vi "SendCmd.vi"(9 "cmd":string, 10 "exe":string="D:\\Program Files\\MVTec\\HALCON-17.12-Progress\\bin\\x64-win64\\hdevelop.exe") -> (0 "error out":errorcluster caption="错误输出", 1 "standard output":string, 2 "return code":i32 caption="返回代码", 3 "standard error":string)   [LabVIEW 2017]
panel:
  out "returnCode":string
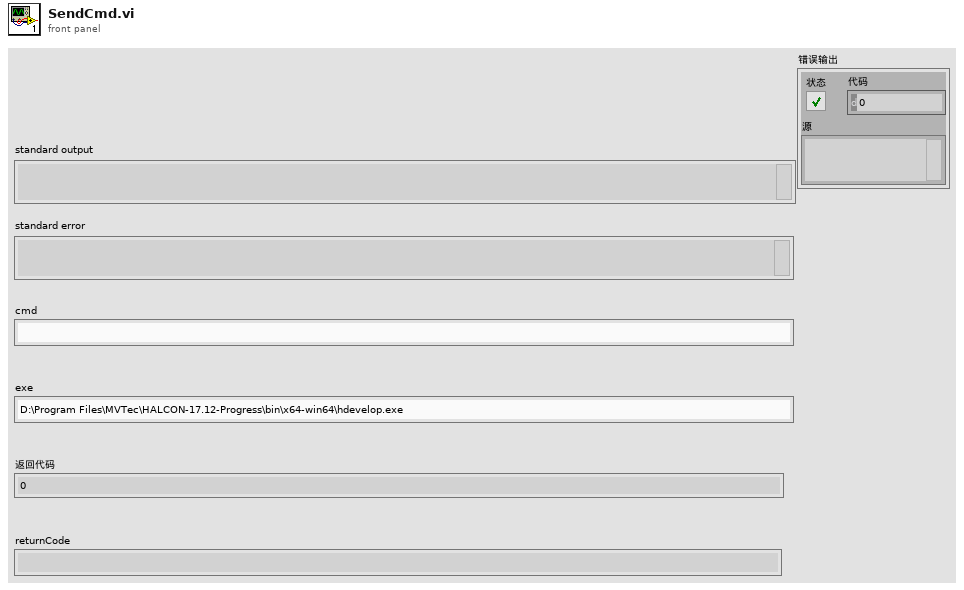
[diagram p1: front panel]
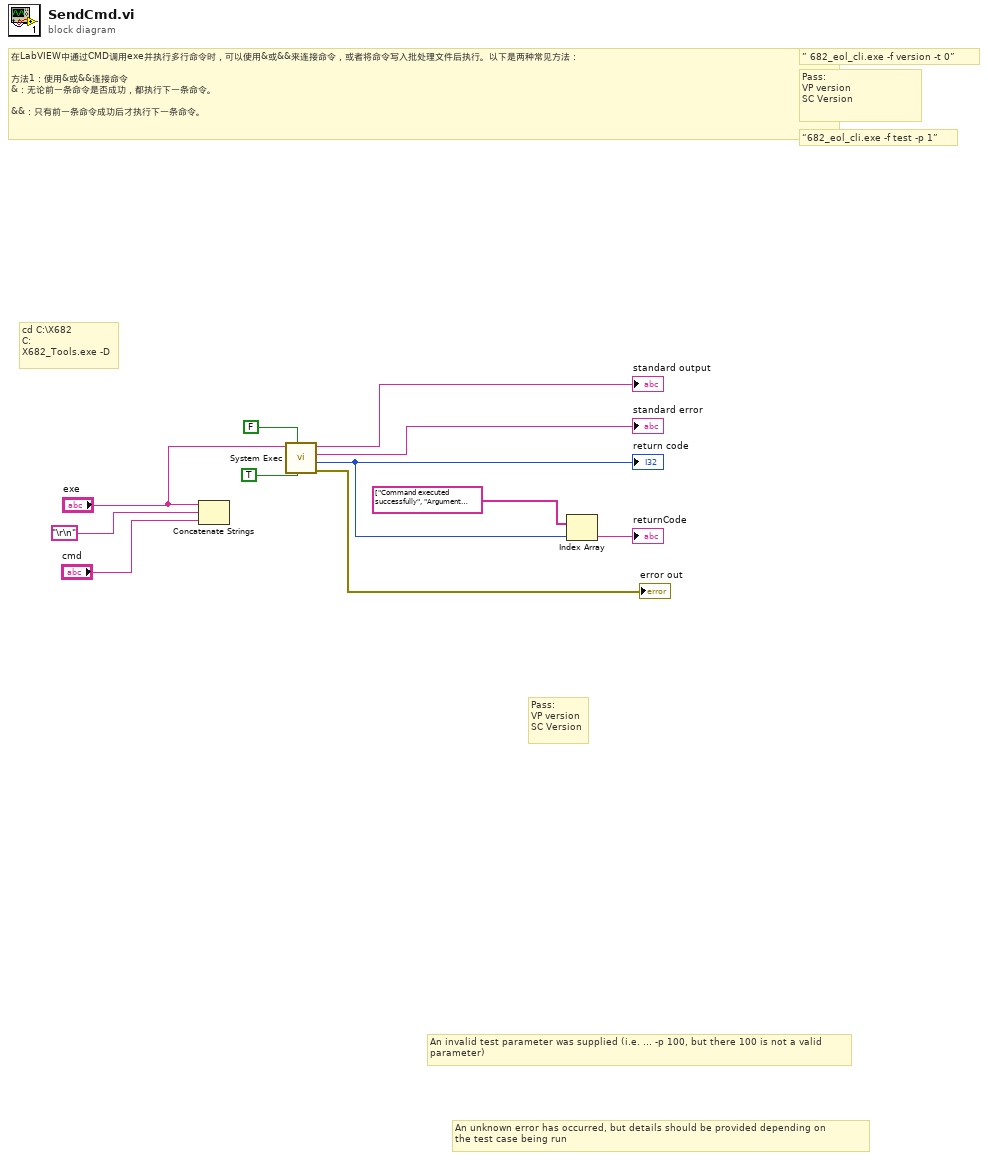
[diagram p0: block diagram]
diagram:
  # "Pass: \nVP version\nSC Version"
  # "cd C:\\X682\nC:\nX682_Tools.exe -D"
  # "An unknown error has occurred, but details should be provided depending on \nthe test case being run"
  # "An invalid test parameter was supplied (i.e. ... -p 100, but there 100 is not a valid \nparameter)"
  # "在LabVIEW中通过CMD调用exe并执行多行命令时，可以使用&或&&来连接命令，或者将命令写入批处理文件后执行。以下是两种常见方法：\n\n方法1：使用&或&&连接命令\n&：无论前一条命令是否成功，都执行下一条命令。\n\n&&：只有前一条命令成功后才执行下一条命令。"
  # "“682_eol_cli.exe -f test -p 1”"
  # "Pass: \nVP version\nSC Version"
  # "” 682_eol_cli.exe -f version -t 0”"
  n1 = Concatenate Strings("exe", "\r\n", "cmd") -> ()  [unwired: 1 out]
  n2 = call <vilib>:"System Exec.vi"("run minimized? (F)"=TRUE, "wait until completion? (T)"=FALSE ("wait until completion?"), "command line"="exe") -> ("error out"=→"error out":errorcluster, "return code"=w3:i32, "standard error"=→"standard error":string, "standard output"=→"standard output":string)  [unwired: 3 in, 2 out]
  "return code" <- w3
  n3 = Index Array(array=string[] ["Command executed successfully", "Argument missing from command line", "An invalid argument wasa provided to command line", "Connection error occurred or no connection", "A message was sent out but did not receive a response in time or there was no response at all\n", "An invalid test parameter was supplied (i.e. ... -p 100, but there 100 is not a valid parameter)\n", "An invalid test parameter was supplied (i.e. ... -p 100, but there 100 is not a valid parameter)", "An unknown error has occurred, but details should be provided depending on the test case being run\n"], index=w3) -> (element=→"returnCode":string)
